vi "Append New Table with Cell Styles.vi"(4 "Row.Headers":string[](array[string]), 6 "Column.Headers":string[](array[string]), 8 "error in (no error)":errorcluster, 9 "Cell.Styles":refnum<class "Style.lvclass">[][](array[class]), 10 "Table.Data":string[][](array[string]), 11 "xwpfDocument in":refnum<class "xwpfDocument.lvclass">) -> (0 "error out":errorcluster, 3 "xwpfDocument out":refnum<class "xwpfDocument.lvclass">)   [LabVIEW 2017, in "Word_Specific.lvlib" / "xwpfDocument.lvclass"]
uses:
  xwpfDocument.lvclass
  Styles/Style/Style.lvclass
  xwpfDocument.lvclass/xwpfDocument.ctl
  C:/Users/Neo/Desktop/Dev_Tools_BR/LabVIEW_NPOI/src/lib/NPOI 2.1.1/NPOI.OOXML.dll
  lib/NPOI 2.1.1/NPOI.OOXML.dll
  xwpfTable/xwpfTable.lvclass
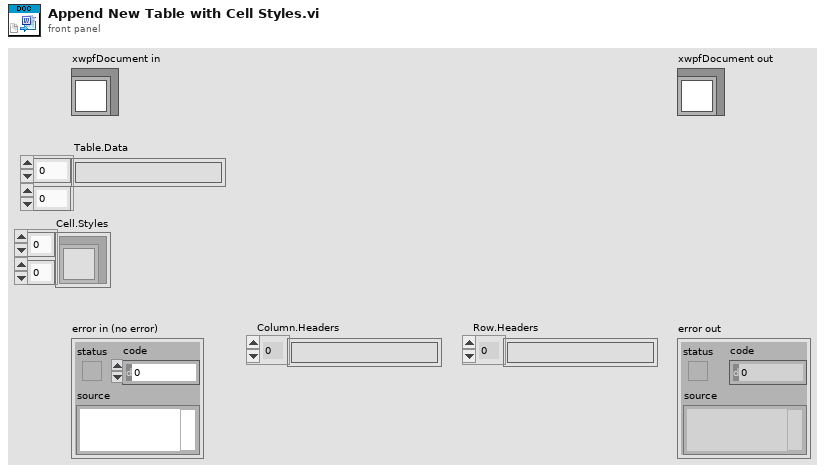
[diagram p1: front panel]
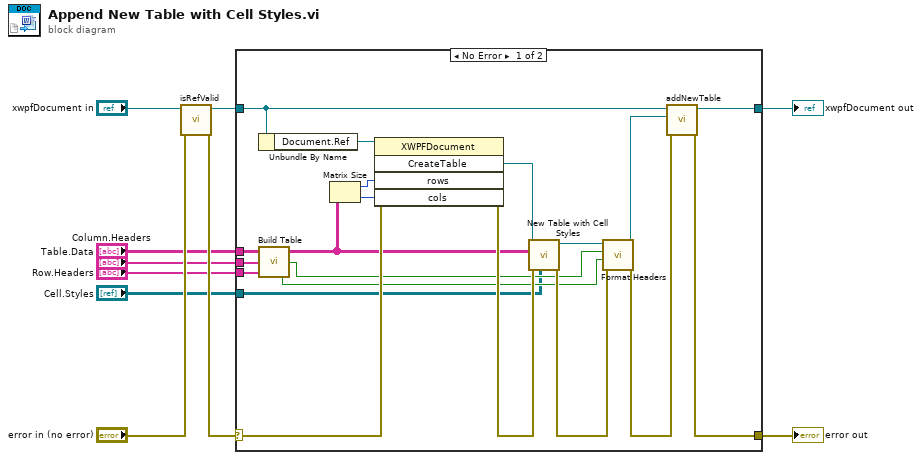
[diagram p0: block diagram]
diagram:
  n1 = call-dynamic "isRefValid.vi"("error in (no error)"="error in (no error)", "xwpfDocument in"="xwpfDocument in") -> ("error out"=w5:errorcluster, "xwpfDocument out"=w7:refnum<class "xwpfDocument.lvclass">)  [unwired: 8 in]
  n2 = case shown="No Error" w5 {
    selector: w5 -> [w25 w32]
    tunnel: [w29 w32] -> w10
    tunnel: [w30 w31] -> w8
    tunnel: w7 -> [w28 w31]
    tunnel: "Table.Data" -> [w21 _]
    tunnel: "Cell.Styles" -> [w11 _]
    tunnel: "Row.Headers" -> [w19 _]
    tunnel: "Column.Headers" -> [w18 _]
    frame No Error {
      n3 = Unbundle By Name(w28) -> ("Document.Ref"=w26:refnum<k24>)
      n4 = call "Build Table.vi"("Row.Headers"=w19, "Column.Headers"=w18, "Table.Data.Text"=w21) -> ("Column.Headers"=w12:bool, "Row.Headers"=w13:bool, "Table.Text"=w20:string[][])
      n5 = Matrix Size(0:w20) -> (1:w24:i32, 2:w23:i32)
      n6 = invoke class="XWPFDocument" method="CreateTable"(reference=w26, error in=w25, "rows"=w24, "cols"=w23) -> (error out=w27:errorcluster, "CreateTable"=w22:refnum<k24>)  [unwired: 1 in, 3 out]
      n7 = call "New Table with Cell Styles.vi"("Cell.Styles"=w11, "error in (no error)"=w27, "Table"=w20, "Table Ref"=w22) -> ("error out"=w15:errorcluster, "xwpfTable out"=w17:refnum<class "xwpfTable.lvclass">)  [unwired: 6 in]
      n8 = call "Format Headers.vi"("error in (no error)"=w15, "Column.Headers"=w12, "Row.Headers"=w13, "xwpfTable in"=w17) -> ("error out"=w14:errorcluster, "xwpfTable out"=w16:refnum<class "xwpfTable.lvclass">)  [unwired: 6 in]
      n9 = call "addNewTable.vi"("error in (no error)"=w14, "New Paragraph"=w16, "xwpfDocument in"=w28) -> ("error out"=w29:errorcluster, "xwpfDocument out"=w30:refnum<class "xwpfDocument.lvclass">)  [unwired: 7 in]
    }
    frame Error {
    }
  }
  "error out" <- w10
  "xwpfDocument out" <- w8
